vi "Update README.vi"() -> ()   [LabVIEW 2014]
uses:
  <userlib>/_OpenG.lib/array/array.llb/Delete Elements from 1D Array (String)__ogtk.vi
  <userlib>/_OpenG.lib/string/string.llb/Trim Whitespace (String Array)__ogtk.vi
panel:
  out "markdown Content":string
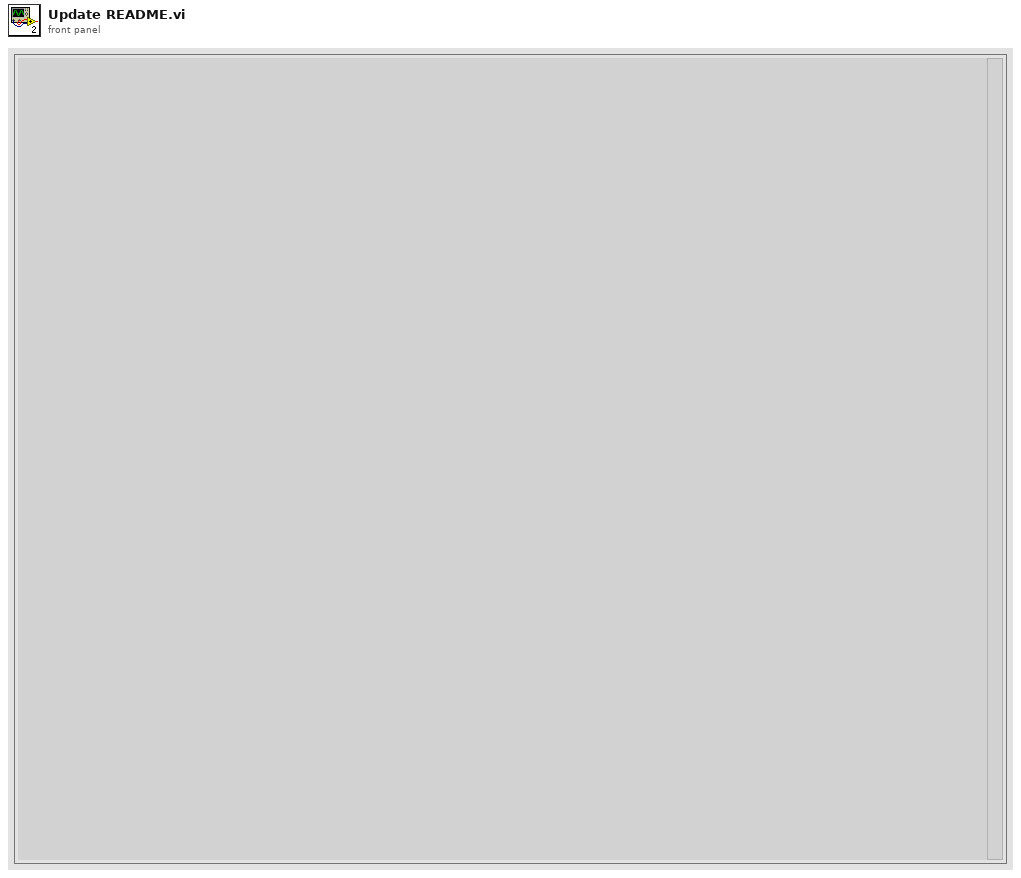
[diagram p1: front panel]
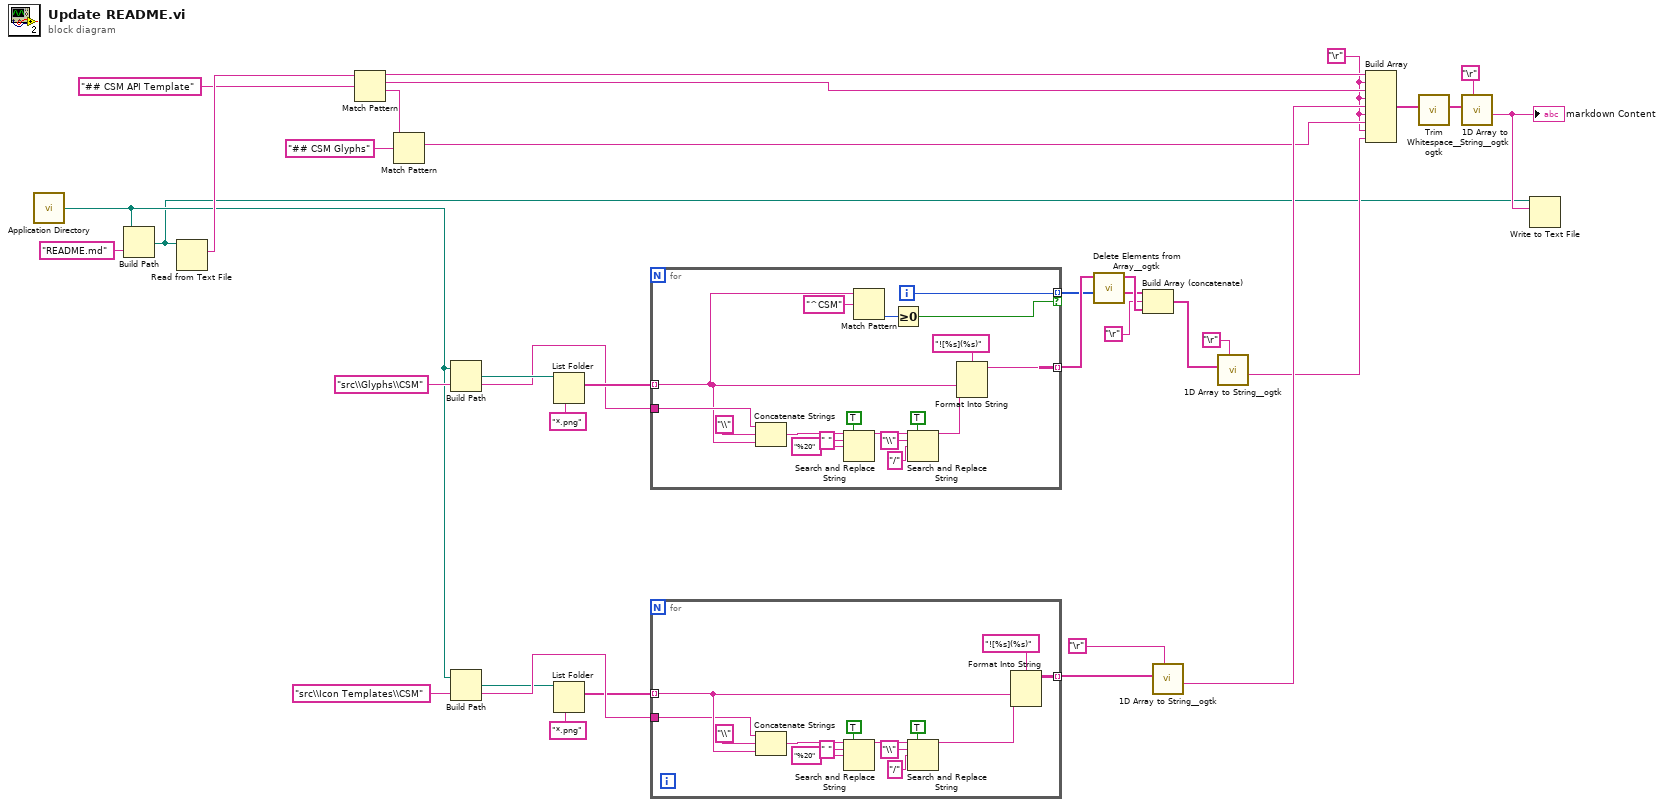
[diagram p0: block diagram]
diagram:
  w11 = "\r"
  w22 = "src\\Icon Templates\\CSM" ("name or relative path")
  w26 = "src\\Glyphs\\CSM" ("name or relative path")
  n1 = call <vilib>:"Application Directory.vi"() -> ("Application Directory"=w9:path)
  n2 = Build Path(base path=w9, name or relative path="README.md") -> (appended path=w7:path)
  n3 = Read from Text File(file (use dialog)=w7) -> (text=w33:string)  [unwired: 3 in, 3 out]
  n4 = Match Pattern(string=w33, regular expression="## CSM API Template") -> (before substring=w18:string, match substring=w17:string, after substring=w32:string)  [unwired: 1 in, 1 out]
  n5 = Match Pattern(string=w32, regular expression="## CSM Glyphs") -> (match substring=w15:string)  [unwired: 1 in, 3 out]
  n6 = Build Path(base path=w9, name or relative path=w26) -> (appended path=w29:path)
  n7 = Build Path(base path=w9, name or relative path=w22) -> (appended path=w19:path)
  n8 = List Folder(path=w29, pattern="*.png") -> (filenames=w27:string[])  [unwired: 2 in, 3 out]
  n9 = List Folder(path=w19, pattern="*.png") -> (filenames=w21:string[])  [unwired: 2 in, 3 out]
  n10 = for {
    tunnel: w27 -> [w39] mode=indexing
    tunnel: w26 -> [w47]
    tunnel: [w46] -> w6 mode=indexing
    tunnel: [w36] -> w5 mode=indexing if=w35
    i -> [w36]
    n11 = Concatenate Strings(w47, "\\" ("string"), w39) -> (w48:string)
    n12 = Search and Replace String(replace all?=TRUE ("replace all? (F)"), input string=w48, search string=" ", replace string="%20" ("replace string (\"\")")) -> (result string=w41:string)  [unwired: 4 in, 3 out]
    n13 = Match Pattern(string=w39, regular expression="^CSM") -> (offset past match=w37:i32)  [unwired: 1 in, 3 out]
    n14 = Greater Or Equal To 0?(x=w37) -> (x >= 0?=w35:bool)
    n15 = Search and Replace String(replace all?=TRUE ("replace all? (F)"), input string=w41, search string="\\", replace string="/" ("replace string (\"\")")) -> (result string=w40:string)  [unwired: 4 in, 3 out]
    n16 = Format Into String(format string="![%s](%s)", w39, w40) -> (resulting string=w46:string)  [unwired: 2 in, 1 out]
  }
  n17 = for {
    tunnel: w21 -> [w65] mode=indexing
    tunnel: w22 -> [w60]
    tunnel: [w59] -> w23 mode=indexing
    n18 = Concatenate Strings(w60, "\\" ("string"), w65) -> (w61:string)
    n19 = Search and Replace String(replace all?=TRUE ("replace all? (F)"), input string=w61, search string=" ", replace string="%20" ("replace string (\"\")")) -> (result string=w54:string)  [unwired: 4 in, 3 out]
    n20 = Search and Replace String(replace all?=TRUE ("replace all? (F)"), input string=w54, search string="\\", replace string="/" ("replace string (\"\")")) -> (result string=w53:string)  [unwired: 4 in, 3 out]
    n21 = Format Into String(format string="![%s](%s)", w65, w53) -> (resulting string=w59:string)  [unwired: 2 in, 1 out]
  }
  n22 = call-poly <userlib>:"Delete Elements from Array__ogtk.vi"("indices"=w5, "array"=w6) -> ("deleted elements"=w3:string[], "array w/ subset deleted"=w4:string[])  [unwired: 8 in]
  n23 = Build Array (concatenate)(w3, "\r", w4) -> (w2:string[])
  n24 = call <userlib>:"1D Array to String__ogtk.vi"("delimiter (Tab)"="\r", "Array of Strings"=w23) -> ("delimited string"=w16:string)  [unwired: 9 in]
  n25 = call <userlib>:"1D Array to String__ogtk.vi"("delimiter (Tab)"="\r", "Array of Strings"=w2) -> ("delimited string"=w14:string)  [unwired: 9 in]
  n26 = Build Array(w18, w11, w17, w11, w16, w11, w15, w11, w14) -> (w12:string[])
  n27 = call-poly <userlib>:"Trim Whitespace__ogtk.vi"("String in"=w12) -> ("String out"=w10:string[])  [unwired: 6 in]
  n28 = call <userlib>:"1D Array to String__ogtk.vi"("delimiter (Tab)"="\r", "Array of Strings"=w10) -> ("delimited string"=w8:string)  [unwired: 9 in]
  "markdown Content" <- w8
  n29 = Write to Text File(file (use dialog)=w7, text=w8) -> ()  [unwired: 2 in, 3 out]
